vi "Add Plugin.vi"(0 "Configuration Session in":refnum<class "Configuration Session.lvclass">, 1 "id":string, 7 "values":T1, 11 "error in (no error)":errorcluster) -> (4 "Configuration Session out":refnum<class "Configuration Session.lvclass">, 6 "exists?":bool, 15 "error out":errorcluster)   [LabVIEW 2017, in "DSF Core.lvlib" / "Configuration Session.lvclass"]
uses:
  Configuration Session.lvclass
  Public/Controls/DSF Plugin Info.ctl
  Public/Controls/DSF Timing Info.ctl
  Public/Controls/DSF Engine Plugin Thread Configuration.ctl
  Public/Controls/DSF Settings Info.ctl
  Configuration Session.lvclass/Configuration Session.ctl
  Controls/DSF File Format/Internal DSF Plugin with ID.ctl
  Controls/DSF File Format/Internal DSF Plugin Info.ctl
  DSF Core.lvlib
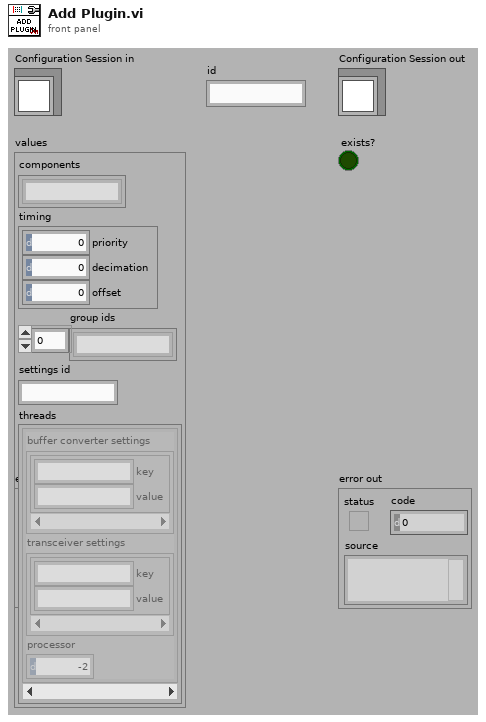
[diagram p1: front panel]
types:
  T1 = typedef "DSF Core.lvlib/DSF Plugin Info.ctl" = cluster{"components":string[], "timing":T2, "group ids":string[], "settings id":string, "threads":T3[]}
  T2 = typedef "DSF Core.lvlib/DSF Timing Info.ctl" = cluster{"priority":u64, "decimation":u64, "offset":u64}
  T3 = typedef "DSF Core.lvlib/DSF Engine Plugin Thread Configuration.ctl" = cluster{"buffer converter settings":T4, "transceiver settings":T4, "processor":i32}
  T4 = typedef "DSF Core.lvlib/DSF Settings Info.ctl" = cluster{"key":string, "value":string}[]
  T5 = typedef "DSF Core.lvlib/Configuration Session.lvclass/Internal DSF Plugin with ID.ctl" = cluster{"id":string, "values":T6}
  T6 = typedef "DSF Core.lvlib/Configuration Session.lvclass/Internal DSF Plugin Info.ctl" = cluster{"components":string[], "timing":T2, "group ids":string[], "settings id":string, "threads":T3[]}
  T7 = typedef "DSF Core.lvlib/Configuration Session.lvclass/DSF Config Data Ref.ctl" = refnum<data-value>
  T8 = typedef "DSF Core.lvlib/Configuration Session.lvclass/DSF Config Data.ctl" = cluster{"dsf configuration":T9, "path":path, "dirty":bool}
  T9 = typedef "DSF Core.lvlib/Configuration Session.lvclass/Internal DSF Configuration.ctl" = cluster{"dsfversion":T10, "version":T10, "plugins":T5[], "groups":T11[], "transfers":T13[], "channels":T15[], "settings":T17[]}
  T10 = typedef "DSF Core.lvlib/DSF Version Info.ctl" = cluster{"major":u32, "minor":u32, "fix":u32, "build":string}
  T11 = typedef "DSF Core.lvlib/Configuration Session.lvclass/Internal DSF Group with ID.ctl" = cluster{"id":string, "values":T12}
  T12 = typedef "DSF Core.lvlib/Configuration Session.lvclass/Internal DSF Group Info.ctl" = cluster{"direction":i32, "timing":T2, "transfer ids":string[], "settings id":string}
  T13 = typedef "DSF Core.lvlib/Configuration Session.lvclass/Internal DSF Transfer with ID.ctl" = cluster{"id":string, "values":T14}
  T14 = typedef "DSF Core.lvlib/Configuration Session.lvclass/Internal DSF Transfer Info.ctl" = cluster{"byte order":i32, "channel ids":string[], "settings id":string}
  T15 = typedef "DSF Core.lvlib/Configuration Session.lvclass/Internal DSF Channel with ID.ctl" = cluster{"id":string, "values":T16}
  T16 = typedef "DSF Core.lvlib/Configuration Session.lvclass/Internal DSF Channel Info.ctl" = cluster{"count":u64, "buffer offset":u64, "data type":i32, "settings id":string}
  T17 = typedef "DSF Core.lvlib/Configuration Session.lvclass/Internal DSF Settings with ID.ctl" = cluster{"id":string, "values":T18}
  T18 = typedef "DSF Core.lvlib/Configuration Session.lvclass/Internal DSF Settings Info.ctl" = cluster{"key":string, "value":string}[]
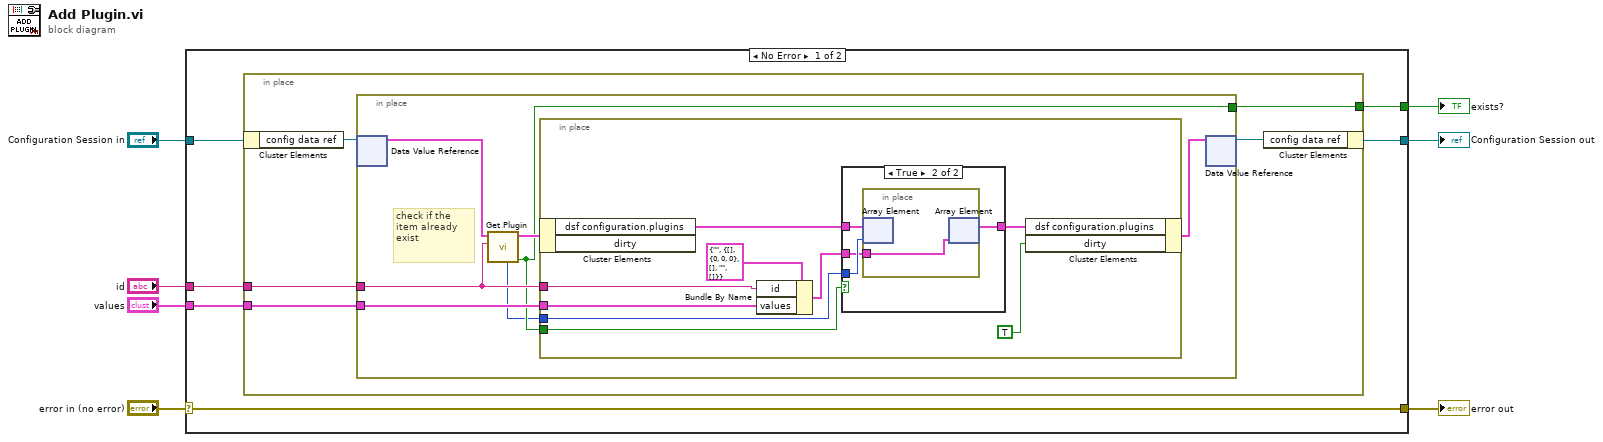
[diagram p0: block diagram]
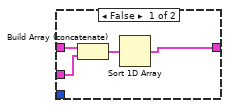
[diagram p2: hidden frame]
diagram:
  n1 = case shown="No Error" "error in (no error)" {
    selector: "error in (no error)" -> [w13 w45]
    tunnel: [w13 w45] -> w6
    tunnel: "id" -> [w12 _]
    tunnel: "values" -> [w11 _]
    tunnel: [w10 _] -> w3
    tunnel: "Configuration Session in" -> [w9 w44]
    tunnel: [w8 w44] -> w1
    frame No Error {
      n2 = in-place {
        in-place-border: w12 -> [w18]
        in-place-border: w11 -> [w17]
        in-place-border: [w16] -> w10
        n3 = in-place-cluster #1(w9) -> ("config data ref"=w15:T7)
        n4 = in-place {
          in-place-border: w18 -> [w25]
          in-place-border: w17 -> [w23]
          in-place-border: [w22] -> w16
          # "check if the item already exist"
          n5 = in-place-dvr #2(w15) -> (w20:T8)  [unwired: 1 out]
          n6 = call "Get Plugin.vi"("id"=w25, "DSF Configuration in"=w20) -> ("exists?"=w22:bool, "DSF Configuration out"=w24:T8, "index"=w21:i32)  [unwired: 7 out]
          n7 = in-place {
            in-place-border: w25 -> [w33]
            in-place-border: w23 -> [w31]
            in-place-border: w22 -> [w30]
            in-place-border: w21 -> [w29]
            n8 = in-place-cluster #3(w24) -> ("dsf configuration.plugins"=w34:T5[])  [unwired: 1 out]
            n9 = Bundle By Name(cluster=T5 {"id"="", "values"={"components"=[], "timing"={"priority"=0, "decimation"=0, "offset"=0}, "group ids"=[], "settings id"="", "threads"=[]}} ("plugin"), "id"=w33, "values"=w31) -> (w27:T5)
            n10 = case shown="True" w30 {
              tunnel: w34 -> [w38 w42]
              tunnel: [w37 w39] -> w32
              tunnel: w29 -> [_ w41]
              tunnel: w27 -> [w35 w40]
              frame False {
                n11 = Build Array (concatenate)(w38, w35) -> (w36:T5[])
                n12 = Sort 1D Array(array=w36) -> (sorted array=w37:T5[])
              }
              frame True {
                n13 = in-place {
                  in-place-border: w40 -> [w43]
                  n14 = in-place-array #4(w42, w41) -> ()  [unwired: 1 out]
                  n15 = in-place-array #4(w43) -> (w39:T5[])  [unwired: 1 out]
                }
              }
            }
            n16 = in-place-cluster #3("dsf configuration.plugins"=w32, "dirty"=TRUE) -> (w19:T8)
          }
          n17 = in-place-dvr #2(w19) -> (w14:T7)  [unwired: 1 out]
        }
        n18 = in-place-cluster #1("config data ref"=w14) -> (w8:refnum<class "Configuration Session.lvclass">)
      }
    }
    frame Error {
    }
  }
  "error out" <- w6
  "exists?" <- w3
  "Configuration Session out" <- w1
